vi "Ensure Dependencies Created.vi"(8 "error in (no error)":errorcluster, 10 "Dependency Name":string, 11 "SMO in":refnum<class "SMO.lvclass">) -> (0 "error out":errorcluster, 2 "Unique Dependency name":string, 3 "SMO out":refnum<class "SMO.lvclass">)   [LabVIEW 2019, in "SMO.lvclass"]
doc: "JKI State Machine Objects (SMO) 1.3.0.56\nJKI - JKI\nCopyright (c) 2017, JKI"
uses:
  SMO.lvclass
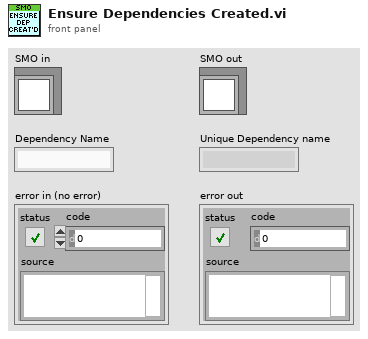
[diagram p1: front panel]
types:
  T1 = typedef "SMO.lvclass/SMOState --Enum.ctl" = enum16{"unknown", "Created", "Started", "Stopped"}
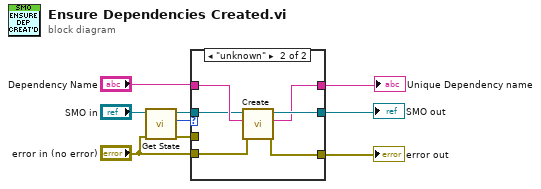
[diagram p0: block diagram]
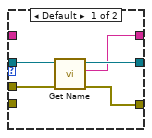
[diagram p2: hidden frame]
diagram:
  n1 = call "Get State.vi"("error in (no error)"="error in (no error)", "SMO"="SMO in") -> ("error out"=w5:errorcluster, "SMO State"=w6:T1, "SMO out"=w4:refnum<class "SMO.lvclass">)  [unwired: 7 in]
  n2 = case shown="\"unknown\"" w6 {
    tunnel: [w11 w15] -> w9
    tunnel: [w12 w20] -> w1
    tunnel: "Dependency Name" -> [_ w19]
    tunnel: [w10 w18] -> w8
    tunnel: w4 -> [w14 w17]
    tunnel: w5 -> [w13 _]
    tunnel: "error in (no error)" -> [_ w16]
    frame Default {
      n3 = call "Get Name.vi"("error in (no error)"=w13, "SMO"=w14) -> ("error out"=w11:errorcluster, "Name"=w10:string, "SMO out"=w12:refnum<class "SMO.lvclass">)  [unwired: 7 in]
    }
    frame "unknown" {
      n4 = call "Create.vi"("error in (no error)"=w16, "Subsystem Name (optional)"=w19, "SMO"=w17) -> ("error out"=w15:errorcluster, "SMO name"=w18:string, "SMO out"=w20:refnum<class "SMO.lvclass">)  [unwired: 6 in]
    }
  }
  "error out" <- w9
  "Unique Dependency name" <- w8
  "SMO out" <- w1
